vi "Switch Shutdown (3706).vi"(8 "error in (no error)":errorcluster, 11 "VISA resource name in":refnum<visa-resource-name>) -> (0 "error out":errorcluster, 3 "VISA resource name out":refnum<visa-resource-name>)   [LabVIEW 2016, in "Hall Effect Library.lvlib"]
uses:
  Hall Effect Library.lvlib
  <instrlib>/Keithley 3706/Keithley 3706.lvlib
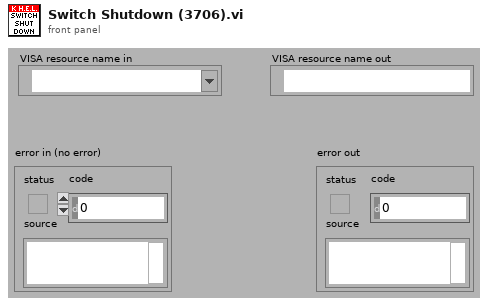
[diagram p1: front panel]
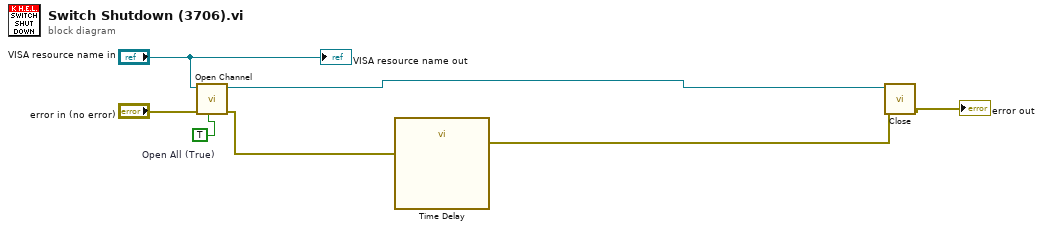
[diagram p0: block diagram]
diagram:
  w7 = TRUE  # Open All (True)
  n1 = call <instrlib>:"Open Channel.vi"("Open All (False)"=w7, "error in (no error)"="error in (no error)", "VISA resource name"="VISA resource name in") -> ("error out"=w3:errorcluster, "VISA resource name out"=w1:refnum<visa-resource-name>)  [unwired: 7 in]
  n2 = call "Time Delay"("error in (no error)"=w3) -> ("error out"=w2:errorcluster)  [unwired: 10 in]
  n3 = call <instrlib>:"Close.vi"("error in (no error)"=w2, "VISA resource name"=w1) -> ("error out"=→"error out":errorcluster)  [unwired: 9 in]
  "VISA resource name out" <- "VISA resource name in"
